vi "ACT_LabVEIW_bartelmmj_conditionalFlow.vi"() -> ()   [LabVIEW 2016]
panel:
  out "?":string
  in  "PH":dbl
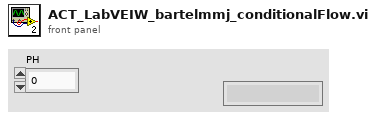
[diagram p1: front panel]
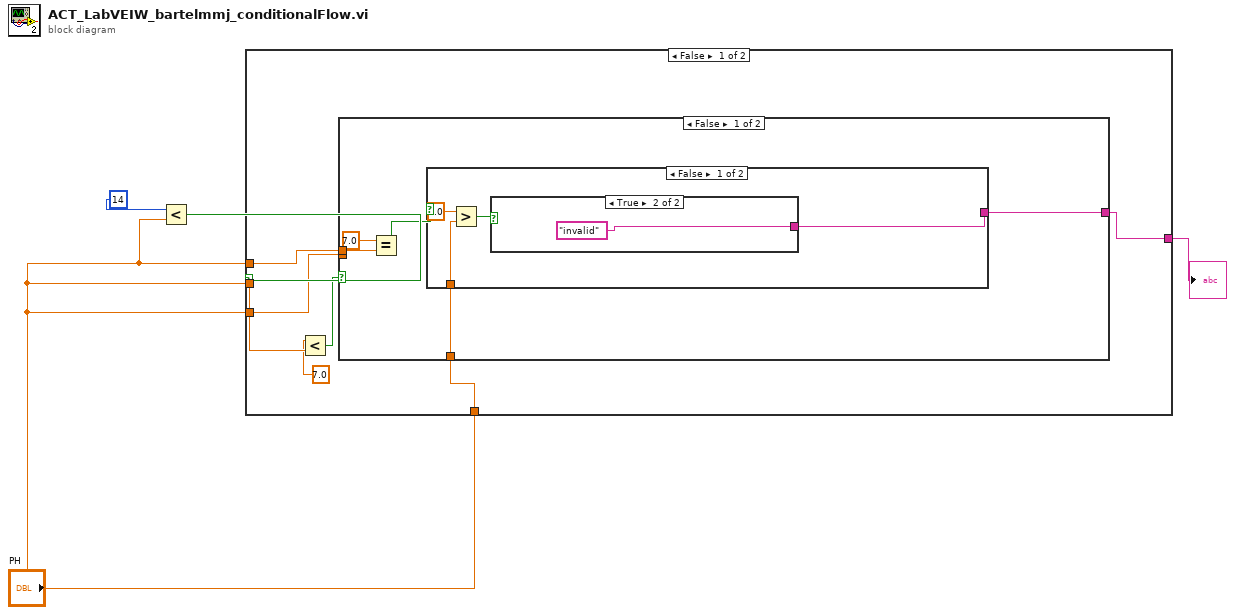
[diagram p0: block diagram]
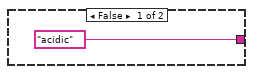
[diagram p2: hidden frame]
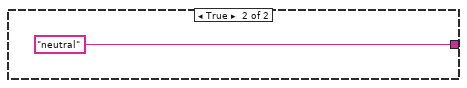
[diagram p3: hidden frame]
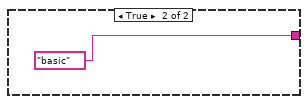
[diagram p4: hidden frame]
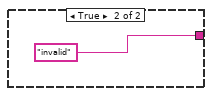
[diagram p5: hidden frame]
diagram:
  n1 = Less?(x=14, y="PH") -> (x < y?=w3:bool)
  n2 = case shown="False" w3 {
    tunnel: [w6 "invalid"] -> w2
    tunnel: "PH" -> [w11 _]
    tunnel: "PH" -> [w9 _]
    tunnel: "PH" -> [w8 _]
    tunnel: "PH" -> [w7 _]
    frame False {
      n3 = Less?(x=7.0, y=w11) -> (x < y?=w5:bool)
      n4 = case shown="False" w5 {
        tunnel: w9 -> [_ _]
        tunnel: w8 -> [w16 _]
        tunnel: [w13 "basic"] -> w6
        tunnel: w7 -> [w12 _]
        frame False {
          n5 = Equal?(x=7.0, y=w16) -> (x = y?=w14:bool)
          n6 = case shown="False" w14 {
            tunnel: [w17 "neutral"] -> w13
            tunnel: w12 -> [w20 _]
            frame False {
              n7 = Greater?(x=0.0, y=w20) -> (0:w18:bool)
              n8 = case shown="True" w18 {
                tunnel: ["acidic" "invalid"] -> w17
                frame False {
                }
                frame True {
                }
              }
            }
            frame True {
            }
          }
        }
        frame True {
        }
      }
    }
    frame True {
    }
  }
  "?" <- w2
